vi "Close.vi"(0 "VisaCluster":T1, 11 "error in (no error)":errorcluster) -> (15 "error out":errorcluster)   [LabVIEW 2014, in "FH 55.lvlib"]
doc: "Performs an instrument error query before terminating the software connection to the instrument."
uses:
  FH 55.lvlib
  TypeDef/VisaCluster.ctl
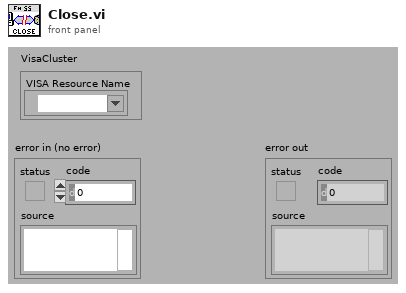
[diagram p1: front panel]
types:
  T1 = typedef "FH 55.lvlib/VisaCluster.ctl" = cluster{"VISA Resource Name":refnum<visa-resource-name>}
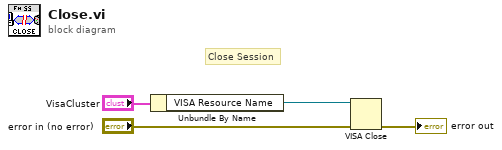
[diagram p0: block diagram]
diagram:
  # "Close Session"
  n1 = Unbundle By Name("VisaCluster") -> ("VISA Resource Name"=w2:refnum<visa-resource-name>)
  n2 = VISA Close(VISA resource name=w2, error in (no error)="error in (no error)") -> (error out=→"error out":errorcluster)
